vi "Convert Channel Selection To String.vi"(4 "Channel Selection":enum32{"A", "B", "AB"}(ring)) -> (1 "Channel Name(s)":string[](array[string]))   [LabVIEW 2020]
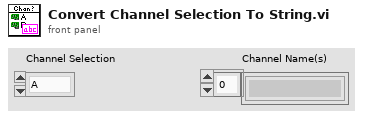
[diagram p1: front panel]
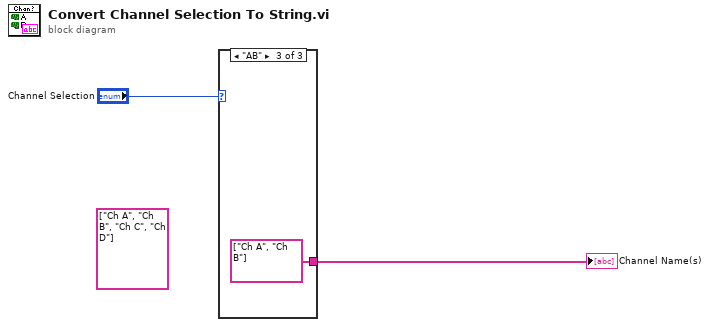
[diagram p0: block diagram]
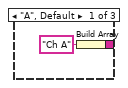
[diagram p2: hidden frame]
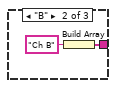
[diagram p3: hidden frame]
diagram:
  (unwired) string[] ["Ch A", "Ch B", "Ch C", "Ch D"]
  n1 = case shown="\"AB\"" "Channel Selection" {
    tunnel: [w3 w6 string[] ["Ch A", "Ch B"]] -> w2
    frame "A", Default {
      n2 = Build Array("Ch A") -> (w3:string[])
    }
    frame "B" {
      n3 = Build Array("Ch B") -> (w6:string[])
    }
    frame "AB" {
    }
  }
  "Channel Name(s)" <- w2
